vi "FlatToRichcif_management_common_TimingStatistics.vi"(5 "OutputClusterType":T1, 11 "InputCluster":T3) -> (3 "OutputCluster":T1)   [LabVIEW 2021, in "CIF_PluginLoader_server.lvlib"]
uses:
  CIF_PluginLoader_server.lvlib
  cif_management_common_TimingStatistics_Flat.ctl
  cif_common_TimingStats_Flat.ctl
  cif_management_common_TimingStatistics.ctl
  cif_common_TimingStats.ctl
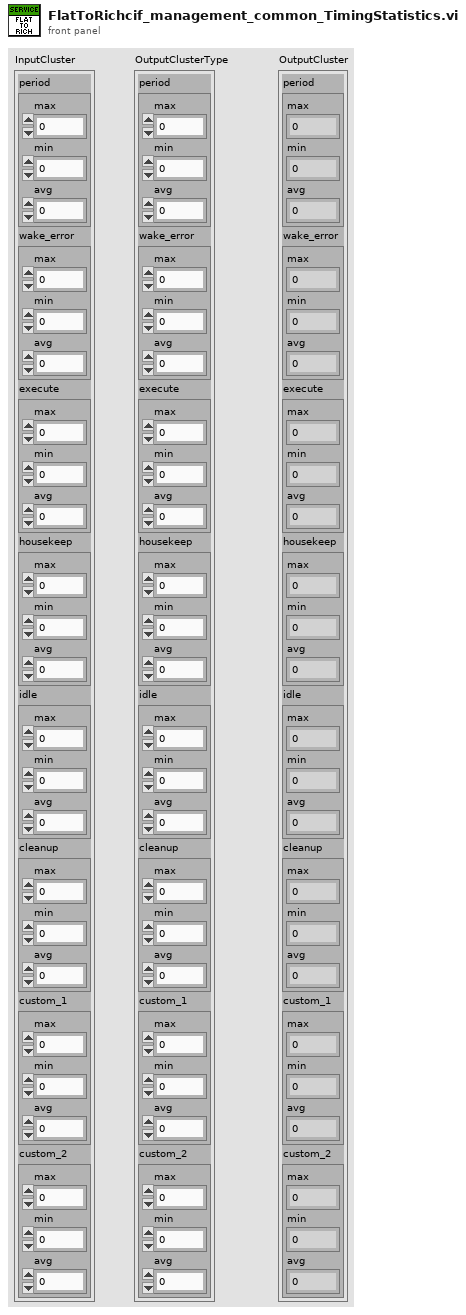
[diagram p1: front panel]
types:
  T1 = typedef "CIF_PluginLoader_server.lvlib/cif_management_common_TimingStatistics.ctl" = cluster{"period":T2, "wake_error":T2, "execute":T2, "housekeep":T2, "idle":T2, "cleanup":T2, "custom_1":T2, "custom_2":T2}
  T2 = typedef "CIF_PluginLoader_server.lvlib/cif_common_TimingStats.ctl" = cluster{"max":i64, "min":i64, "avg":dbl}
  T3 = typedef "CIF_PluginLoader_server.lvlib/cif_management_common_TimingStatistics_Flat.ctl" = cluster{"period":T4, "wake_error":T4, "execute":T4, "housekeep":T4, "idle":T4, "cleanup":T4, "custom_1":T4, "custom_2":T4}
  T4 = typedef "CIF_PluginLoader_server.lvlib/cif_common_TimingStats_Flat.ctl" = cluster{"max":i64, "min":i64, "avg":dbl}
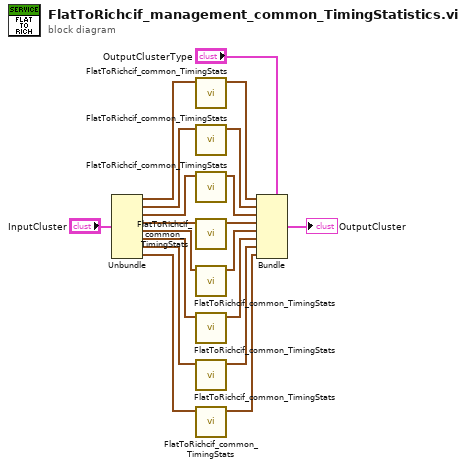
[diagram p0: block diagram]
diagram:
  n1 = Unbundle "Unbundle"("InputCluster") -> ("period"=w16:T4, "wake_error"=w14:T4, "execute"=w12:T4, "housekeep"=w10:T4, "idle"=w8:T4, "cleanup"=w6:T4, "custom_1"=w4:T4, "custom_2"=w2:T4)
  n2 = call "FlatToRichcif_common_TimingStats.vi"("InputCluster"=w16) -> ("OutputCluster"=w15:T2)  [unwired: 10 in]
  n3 = call "FlatToRichcif_common_TimingStats.vi"("InputCluster"=w14) -> ("OutputCluster"=w13:T2)  [unwired: 10 in]
  n4 = call "FlatToRichcif_common_TimingStats.vi"("InputCluster"=w12) -> ("OutputCluster"=w11:T2)  [unwired: 10 in]
  n5 = call "FlatToRichcif_common_TimingStats.vi"("InputCluster"=w10) -> ("OutputCluster"=w9:T2)  [unwired: 10 in]
  n6 = call "FlatToRichcif_common_TimingStats.vi"("InputCluster"=w8) -> ("OutputCluster"=w7:T2)  [unwired: 10 in]
  n7 = call "FlatToRichcif_common_TimingStats.vi"("InputCluster"=w6) -> ("OutputCluster"=w5:T2)  [unwired: 10 in]
  n8 = call "FlatToRichcif_common_TimingStats.vi"("InputCluster"=w4) -> ("OutputCluster"=w3:T2)  [unwired: 10 in]
  n9 = call "FlatToRichcif_common_TimingStats.vi"("InputCluster"=w2) -> ("OutputCluster"=w1:T2)  [unwired: 10 in]
  n10 = Bundle "Bundle"(cluster="OutputClusterType", "period"=w15, "wake_error"=w13, "execute"=w11, "housekeep"=w9, "idle"=w7, "cleanup"=w5, "custom_1"=w3, "custom_2"=w1) -> (→"OutputCluster":T1)
